vi "FindRowIndex.vi"(8 "error in (no error)":errorcluster, 9 "PartNumberData":T1(array[cluster]), 10 "Barcode":string) -> (0 "error out":errorcluster, 1 "SerialNumber":string, 2 "PartNumber":string, 3 "ArrayIndex":i32, 5 "Revision":string)   [LabVIEW 2021]
uses:
  <vilib>/regexp/Match Regular Expression.xnode
panel:
  out "PN_SN":string
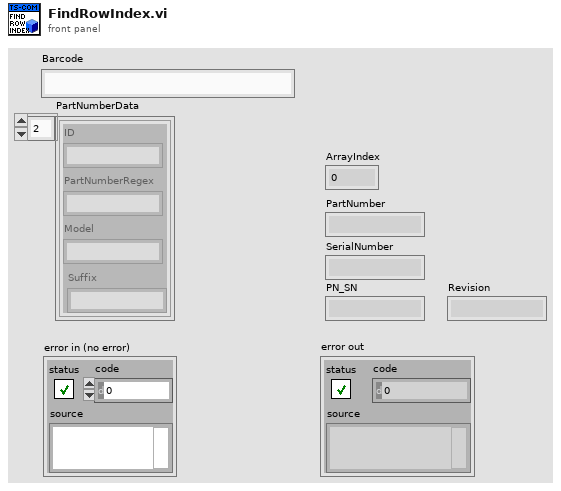
[diagram p1: front panel]
types:
  T1 = cluster{"ID":string, "PartNumberRegex":string, "Model":string, "Suffix":string}[]
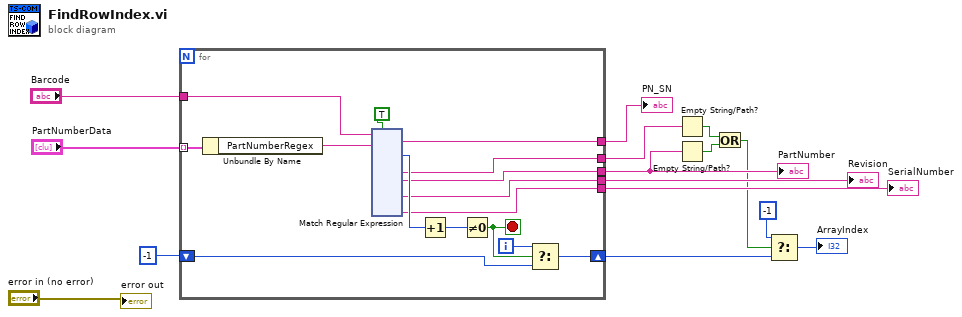
[diagram p0: block diagram]
diagram:
  n1 = for {
    tunnel: "Barcode" -> [w27]
    shift-right: [w23] -> w3
    shift-left: -1 -> [w24]
    tunnel: "PartNumberData" -> [w22] mode=indexing
    tunnel: [w19] -> w7
    tunnel: [w17] -> w11
    tunnel: [w20] -> w10
    tunnel: [w18] -> w9
    tunnel: [w16] -> w8
    i -> [w25]
    stop <- w26 stop-if-true
    n2 = Unbundle By Name(w22) -> ("PartNumberRegex"=w21:string)
    n3 = xnode "Match Regular Expression"("input string"=w27, "regular expression"=w21, "ignore case? (F)"=TRUE) -> ("whole match"=w20:string, "offset past match"=w30:i32, "submatch 1"=w16:string, "submatch 2"=w19:string, "submatch 4"=w18:string, "submatch 6"=w17:string)  [unwired: 3 in, 5 out]
    n4 = Increment(x=w30) -> (x+1=w29:i32)
    n5 = Not Equal To 0?(x=w29) -> (x != 0?=w26:bool)
    n6 = Select(t=w25, s=w26, f=w24) -> (s? t:f=w23:i32)
  }
  "PartNumber" <- w7
  "SerialNumber" <- w11
  "PN_SN" <- w10
  "Revision" <- w9
  n7 = Empty String/Path?(string/path=w8) -> (empty?=w6:bool)
  n8 = Empty String/Path?(string/path=w7) -> (empty?=w5:bool)
  n9 = Or(x=w6, y=w5) -> (x .or. y?=w4:bool)
  n10 = Select(t=-1, s=w4, f=w3) -> (s? t:f=→"ArrayIndex":i32)
  "error out" <- "error in (no error)"
